vi "Bounds.vi"(1 "XRef":refnum<vi>, 2 "State In":T2={"Input Type"=variant(path path ""), "Terminals"=[]}) -> (0 "Bounds":cluster{"Width":T1, "Height":T1})   [LabVIEW 2015, in "Await.xnode"]
doc: "This ability VI is used to tell LabVIEW your current bounds. If you want to update your bounds, you must inform LabVIEW through the UpdateImageAndBounds reply of another ability VI. If you change your bounds, you will also probably want to update your image.\n\nDefault behavior: None.\n\nThis ability does not provide UI and OS messages are not handled."
uses:
  Await.xnode
  State.ctl
  <vilib>/XNodeSupport/XNodeInt.ctl
  <vilib>/XNodeSupport/NI_XNodeSupport.lvlib
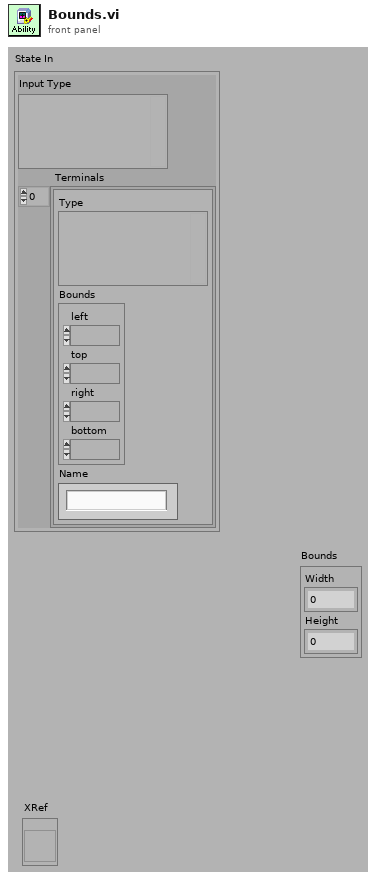
[diagram p1: front panel]
types:
  T1 = typedef "NI_XNodeSupport.lvlib/XNodeInt.ctl" = i32
  T2 = typedef "Await.xnode/State.ctl" = cluster{"Input Type":variant, "Terminals":cluster{"Type":variant, "Bounds":cluster{"left":i16, "top":i16, "right":i16, "bottom":i16}, "Name":string}[]}
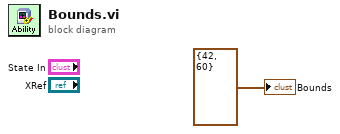
[diagram p0: block diagram]
diagram:
  "Bounds" <- cluster{"Width":T1, "Height":T1} {"Width"=42, "Height"=60} ("Bounds")
